vi "Write CSV File_LV2012_NI_Verified.vi"() -> ()   [LabVIEW 2019]
doc: "This example shows how to use the Write to Spreadsheet VI to write data to a Comma Separated Value (CSV) spreadsheet file which can be read in Microsoft Excel."
uses:
  <vilib>/Utility/file.llb/Write Delimited Spreadsheet (string).vi
  <vilib>/Utility/file.llb/Write Delimited Spreadsheet (DBL).vi
panel:
  out "path":path
  out "error out":errorcluster
  in  "Channel Names":string[](array[string])=["Channel 1", "Channel 2", "Channel 3", "Channel 4", "Channel 5"]
  in  "Header Info":string[][](array[string])=[["Test Name", "Operator", "UUT"], ["Voltage", "National Instruments", "AA123"]]
  in  "Values to Write":i32=20
  in  "stop":bool
  in  "# of Channels":i32=5
  # "Overview: This example shows how to use the Write to Spreadsheet VI to write data to a Comma Separated Value (CSV) spreadsheet file which can be read in Microsoft Excel. \nRequirements: LabVIEW 2012 (or compatible)\nInstructions:\n1.  Choose where you would like to store the file\n2. Write the file properties such as the file header and the channel names\n3. Configure the number of channels and the number of samples/channel you want to generate\n4. Run the VI"
  # "File Properties"
  # "Generate Data"
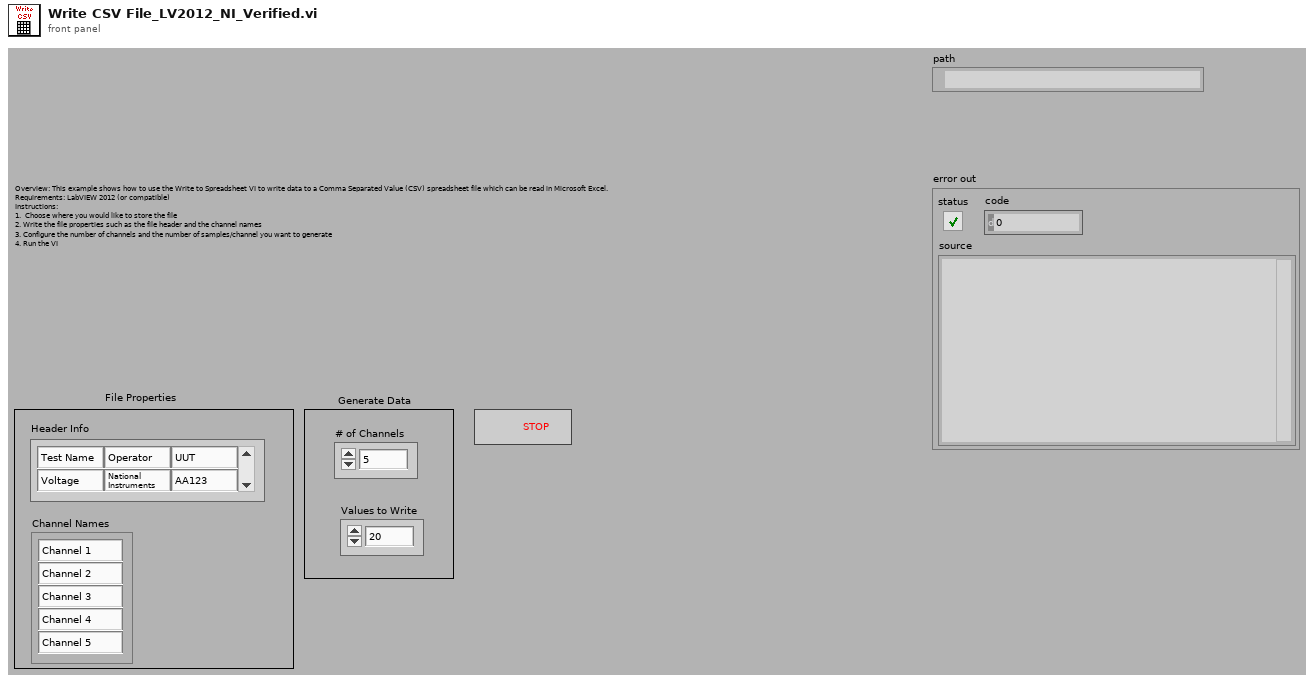
[diagram p1: front panel]
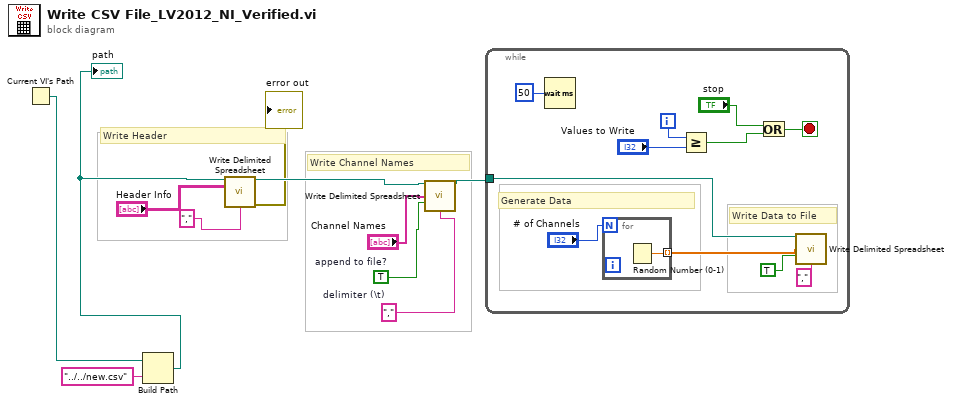
[diagram p0: block diagram]
diagram:
  w6 = TRUE  # append to file?
  w5 = ","  # delimiter (\t)
  # "Write Header"
  # "Write Channel Names"
  n1 = Current VI's Path() -> (path=w3:path)
  n2 = Build Path(base path=w3, name or relative path="../../new.csv") -> (appended path=w1:path)
  "path" <- w1
  n3 = call-poly <vilib>:"Write Delimited Spreadsheet.vi"("file path (dialog if empty)"=w1, "2D data"="Header Info", "delimiter (\\t)"="," ("delimiter (\\t)")) -> ("new file path (Not A Path if cancelled)"=w9:path, "error out"=→"error out":errorcluster)  [unwired: 11 in]
  n4 = call-poly <vilib>:"Write Delimited Spreadsheet.vi"("file path (dialog if empty)"=w9, "1D data"="Channel Names", "append to file? (new file:F)"=w6, "delimiter (\\t)"=w5) -> ("new file path (Not A Path if cancelled)"=w8:path)  [unwired: 10 in, 1 out]
  n5 = while {
    tunnel: w8 -> [w13]
    i -> [w19]
    stop <- w16 stop-if-true
    # "Write Data to File"
    # "Generate Data"
    n6 = Wait (ms)(milliseconds to wait=u32 50 ("millisecond multiple")) -> ()  [unwired: 1 out]
    n7 = for {
      N: "# of Channels" -> [_]
      tunnel: [w23] -> w12 mode=indexing
      n8 = Random Number (0-1)() -> (number: 0 to 1=w23:dbl)
    }
    n9 = Greater Or Equal?(x=w19, y="Values to Write") -> (x >= y?=w17:bool)
    n10 = Or(x="stop", y=w17) -> (x .or. y?=w16:bool)
    n11 = call-poly <vilib>:"Write Delimited Spreadsheet.vi"("file path (dialog if empty)"=w13, "1D data"=w12, "append to file? (new file:F)"=TRUE, "delimiter (\\t)"="," ("delimiter (\\t)")) -> ()  [unwired: 10 in, 2 out]
  }
